vi "ShockTestImpedance_V1.vi"() -> ()   [LabVIEW 2021]
panel:
  out "x > 0? 2":bool
  out "x > 0?":bool
  out "return count":u32
  out "error out":errorcluster
  out "VISA resource name out":refnum<visa-resource-name>
  out "current sample":string
  out "data":dynamicdata(graph)
  in  "error in (no error)":errorcluster
  in  "VISA resource name":refnum<visa-resource-name>
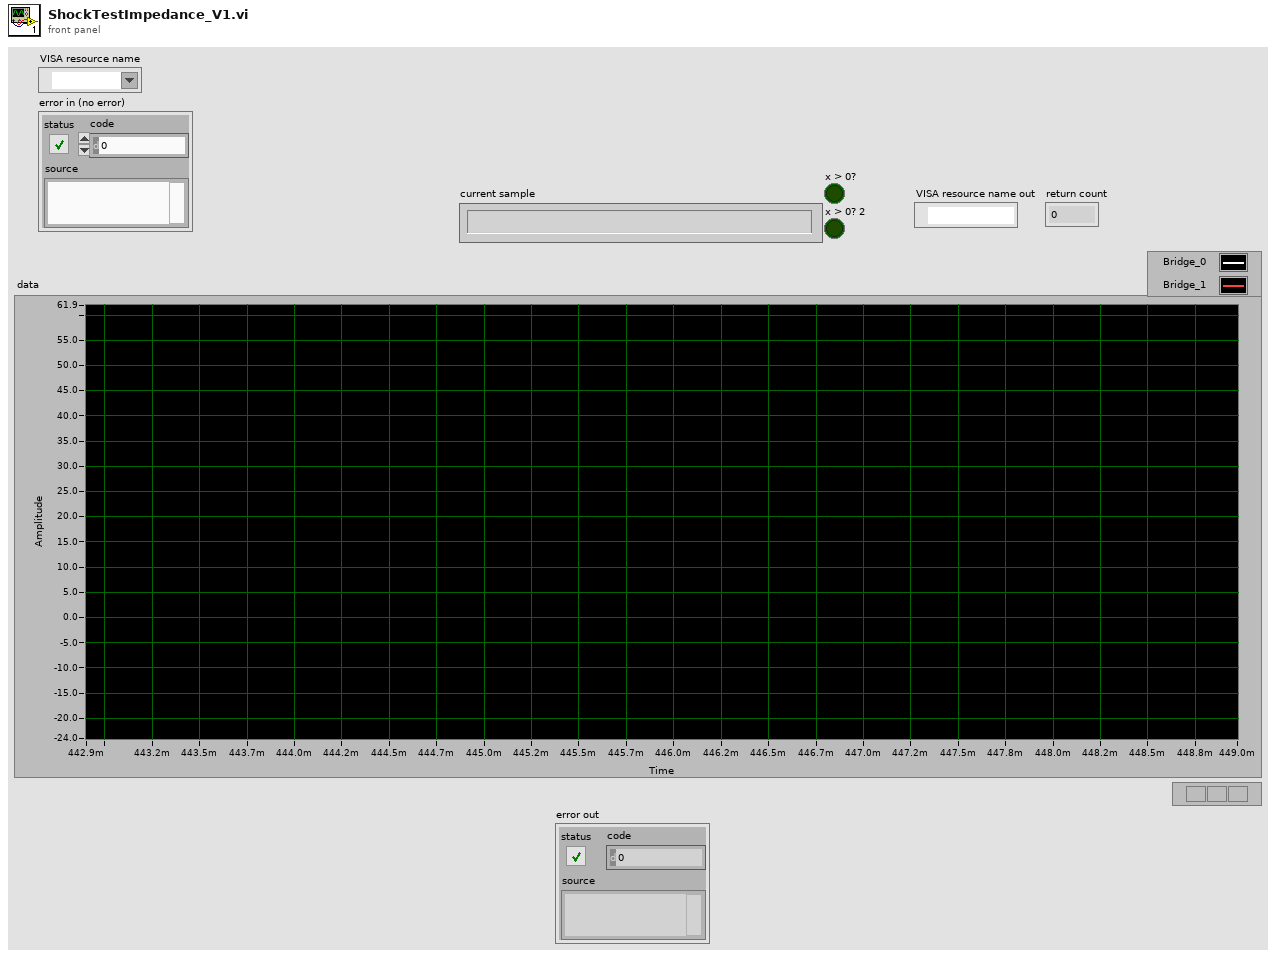
[diagram p1: front panel]
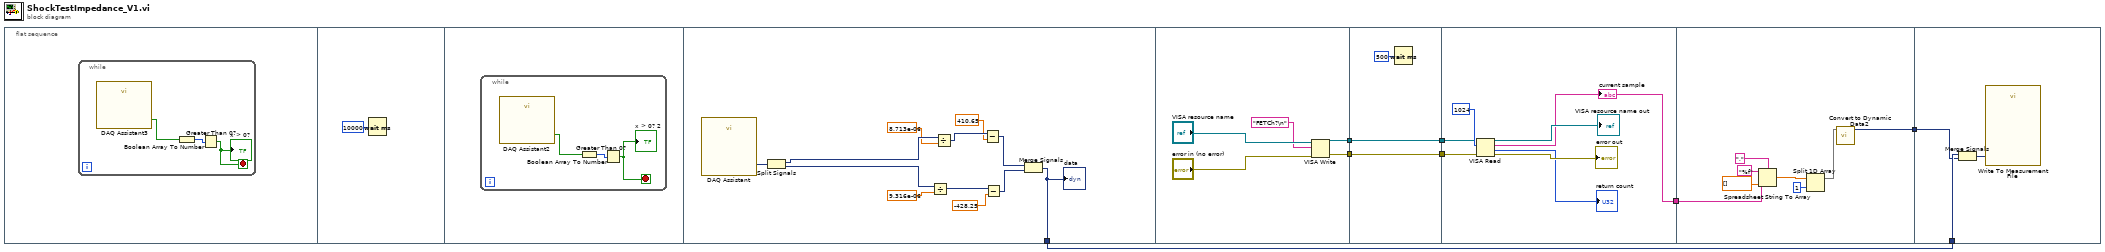
[diagram p0: block diagram]
diagram:
  n1 = flat-sequence {
    tunnel: [w15] -> w1
    tunnel: [w28] -> w7
    tunnel: [w27] -> w6
    tunnel: w7 -> [w34]
    tunnel: w6 -> [w33]
    tunnel: [w34] -> w5
    tunnel: [w33] -> w4
    tunnel: w5 -> [w36]
    tunnel: w4 -> [w37]
    tunnel: [w35] -> w3
    tunnel: w3 -> [w44]
    tunnel: [w42] -> w2
    tunnel: w2 -> [w50]
    tunnel: w1 -> [w51]
    frame #0 {
      n2 = while {
        stop <- w8 stop-if-true
        n3 = call "DAQ Assistant3"() -> ("data"=w10:bool[])  [unwired: 17 in, 2 out]
        n4 = Boolean Array To Number(Boolean array=w10) -> (number=w9:u32)
        n5 = Greater Than 0?(x=w9) -> (x > 0?=w8:bool)
        "x > 0?" <- w8
      }
    }
    frame #1 {
      n6 = Wait (ms)(milliseconds to wait=u32 10000) -> ()  [unwired: 1 out]
    }
    frame #2 {
      n7 = while {
        stop <- w12 stop-if-true
        n8 = call "DAQ Assistant2"() -> ("data"=w14:bool[])  [unwired: 17 in, 2 out]
        n9 = Boolean Array To Number(Boolean array=w14) -> (number=w13:u32)
        n10 = Greater Than 0?(x=w13) -> (x > 0?=w12:bool)
        "x > 0? 2" <- w12
      }
    }
    frame #3 {
      n11 = call "DAQ Assistant"() -> ("data"=w20:dynamicdata)  [unwired: 17 in, 2 out]
      n12 = Split Signals(w20) -> (w25:dynamicdata, w26:dynamicdata)  [unwired: 2 in]
      n13 = Divide(x=w26, y=9.316e-06) -> (x/y=w24:dynamicdata)
      n14 = Divide(x=w25, y=8.713e-06) -> (x/y=w23:dynamicdata)
      n15 = Subtract(x=w23, y=410.65) -> (x-y=w21:dynamicdata)
      n16 = Subtract(x=w24, y=-428.25) -> (x-y=w22:dynamicdata)
      n17 = Merge Signals(w21, w22) -> (w15:dynamicdata)
      "data" <- w15
    }
    frame #4 {
      n18 = VISA Write(VISA resource name="VISA resource name", write buffer="FETCh?\n" ("Command"), error in (no error)="error in (no error)") -> (VISA resource name out=w27:refnum<visa-resource-name>, error out=w28:errorcluster)  [unwired: 1 out]
    }
    frame #5 {
      n19 = Wait (ms)(milliseconds to wait=u32 500 ("delay before read (ms)")) -> ()  [unwired: 1 out]
    }
    frame #6 {
      n20 = VISA Read(VISA resource name=w37, byte count=u32 1024, error in (no error)=w36) -> (VISA resource name out=→"VISA resource name out":refnum<visa-resource-name>, read buffer=w35:string, return count=→"return count":u32, error out=→"error out":errorcluster)
      "current sample" <- w35
    }
    frame #7 {
      n21 = Spreadsheet String To Array(delimiter (Tab)=",", format string="%f", spreadsheet string=w44, array type (2D Dbl)=dbl[] []) -> (array=w48:dbl[])
      n22 = Split 1D Array(array=w48, index=1) -> (first subarray=w49:dbl[])  [unwired: 1 out]
      n23 = call "Convert to Dynamic Data2"("Array"=w49) -> ("Dynamic Data Type"=w42:dynamicdata)  [unwired: 3 in]
    }
    frame #8 {
      n24 = Merge Signals(w51, w50) -> (w52:dynamicdata)
      n25 = call "Write To Measurement File"("Signals"=w52) -> ()  [unwired: 16 in, 3 out]
    }
  }
